vi "Play with cosine waves.vi"() -> ()   [LabVIEW 2024]
uses:
  <vilib>/express/express analysis/Spectral/Block/exnSpectralBlock spectral measurements RMS poly.vi
  <vilib>/express/express analysis/Spectral/Block/exnSpectralBlock spectral measurements RMS WFM.vi
  <vilib>/express/express analysis/Spectral/XNode/ExpressSpectralMeasurementsBlockNode.xnode
panel:
  out "Phase":cluster{"f0":dbl, "df":dbl, "phase":dbl[]}(graph)={"f0"=0.0, "df"=1.0000000000000002, "phase"=array[22000 elements]}
  out "FFT - (RMS)":cluster{"f0":dbl, "df":dbl, "magnitude":dbl[]}(graph)={"f0"=0.0, "df"=1.0000000000000002, "magnitude"=array[22000 elements]}
  out "Waveform Graph":waveform(dbl)(graph)
  in  "Array":T1(array[cluster])=[{"Freq"=440.0, "phase"=0.0, "amplitude"=1.0, "damping factor"=0.0}, {"Freq"=880.0, "phase"=180.0, "amplitude"=0.2, "damping factor"=0.0}, {"Freq"=1760.0, "phase"=94.54545454545455, "amplitude"=0.1, "damping factor"=0.0}] {"phase" scale=0.0..180.0; "Freq" scale=1.0..1000.0}
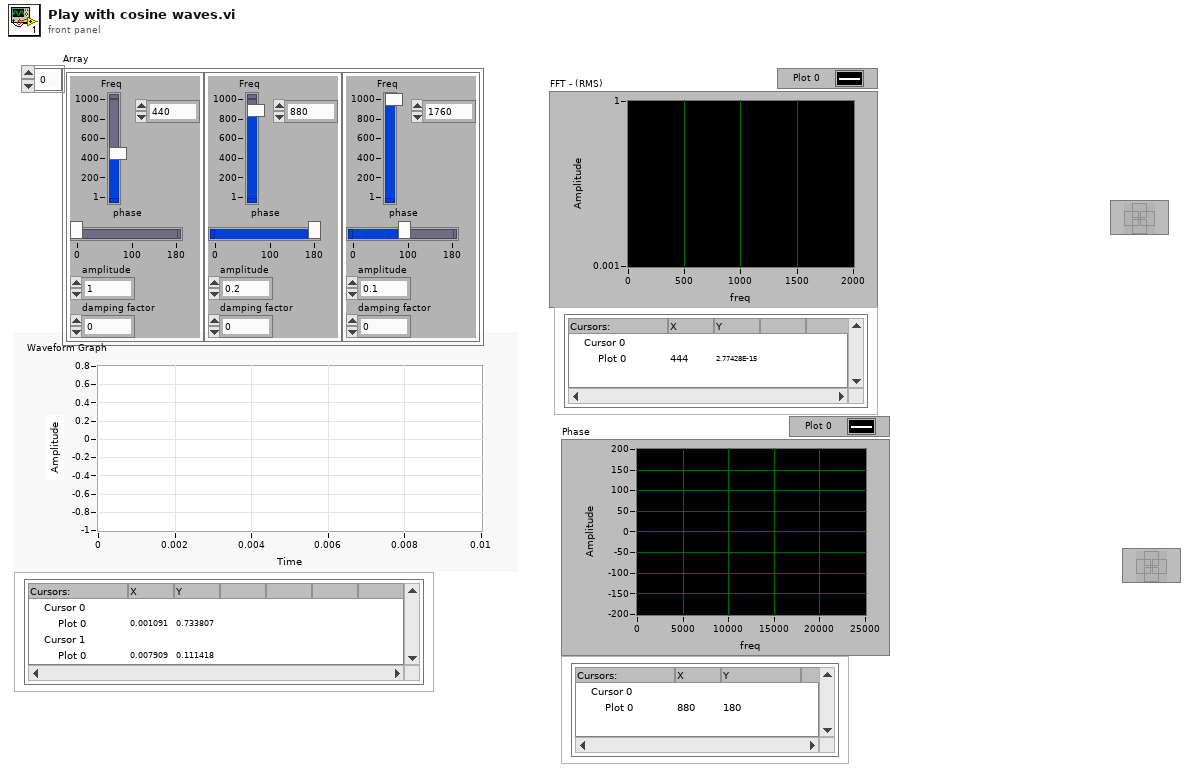
[diagram p1: front panel]
types:
  T1 = cluster{"Freq":dbl, "phase":dbl, "amplitude":dbl, "damping factor":dbl}[]
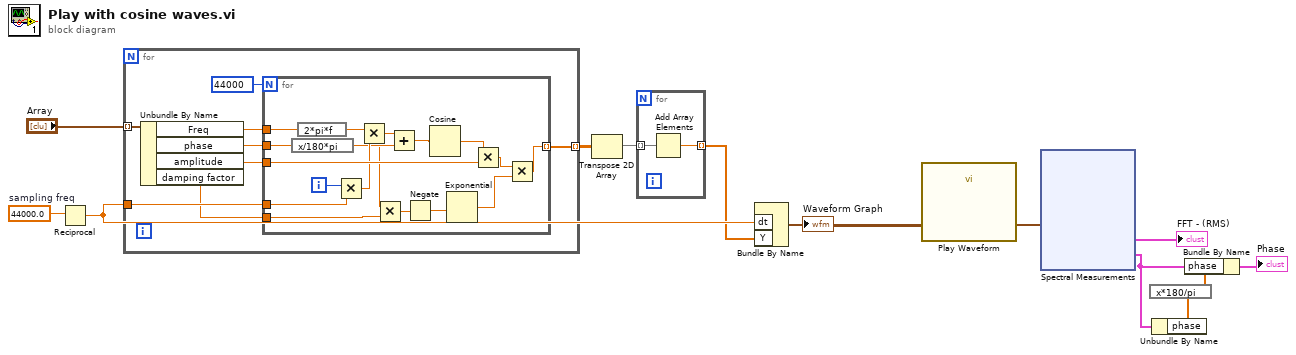
[diagram p0: block diagram]
diagram:
  w11 = 44000.0  # sampling freq
  n1 = Reciprocal(x=w11) -> (1/x=w10:dbl)
  n2 = for {
    tunnel: "Array" -> [w20] mode=indexing
    tunnel: w10 -> [w16]
    tunnel: [w15] -> w9 mode=indexing
    n3 = Unbundle By Name(w20) -> ("Freq"=w18:dbl, "phase"=w17:dbl, "amplitude"=w14:dbl, "damping factor"=w13:dbl)
    n4 = for {
      N: 44000 -> [_]
      tunnel: w18 -> [w37]
      tunnel: w17 -> [w35]
      tunnel: [w23] -> w15 mode=indexing
      tunnel: w16 -> [w32]
      tunnel: w14 -> [w30]
      tunnel: w13 -> [w29]
      i -> [w33]
      n5 = expression code="x/180*pi"(w35) -> (w22:dbl)
      n6 = expression code="2*pi*f"(w37) -> (w36:dbl)
      n7 = Multiply(x=w33, y=w32) -> (x*y=w28:dbl)
      n8 = Multiply(x=w36, y=w28) -> (x*y=w21:dbl)
      n9 = Multiply(x=w21, y=w29) -> (x*y=w27:dbl)
      n10 = Add(x=w21, y=w22) -> (x+y=w34:dbl)
      n11 = Negate(x=w27) -> (-x=w26:dbl)
      n12 = Cosine(x=w34) -> (cos(x)=w31:dbl)
      n13 = Exponential(1:w26) -> (0:w24:dbl)
      n14 = Multiply(x=w31, y=w30) -> (x*y=w25:dbl)
      n15 = Multiply(x=w25, y=w24) -> (x*y=w23:dbl)
    }
  }
  n16 = Transpose 2D Array(2D array=w9) -> (transposed array=w8:dbl[][])
  n17 = for {
    tunnel: w8 -> [w39] mode=indexing
    tunnel: [w38] -> w7 mode=indexing
    n18 = Add Array Elements(numeric array=w39) -> (sum=w38:dbl)
  }
  n19 = Bundle By Name("dt"=w10, "Y"=w7) -> (w1:waveform(dbl))  [unwired: 1 in]
  "Waveform Graph" <- w1
  n20 = call "Play Waveform"("Data"=w1) -> ()  [unwired: 18 in, 1 out]
  n21 = xnode "Spectral Measurements"("Signals"=w1) -> ("FFT - (RMS)"=→"FFT - (RMS)":cluster{"f0":dbl, "df":dbl, "magnitude":dbl[]}, "Phase"=w3:cluster{"f0":dbl, "df":dbl, "phase":dbl[]})  [unwired: 1 in, 1 out]
  n22 = Unbundle By Name(w3) -> ("phase"=w5:dbl[])
  n23 = expression code="x*180/pi"(w5) -> (w4:dbl[])
  n24 = Bundle By Name(cluster=w3, "phase"=w4) -> (→"Phase":cluster{"f0":dbl, "df":dbl, "phase":dbl[]})
